vi "Close.vi"(8 "error in":errorcluster, 11 "lia host in":refnum<class "LIA Host Interface.lvclass">) -> (0 "error out":errorcluster, 3 "lia host out":refnum<class "LIA Host Interface.lvclass">)   [LabVIEW 2017, in "LIA Host Interface.lvclass"]
uses:
  LIA Host Interface.lvclass
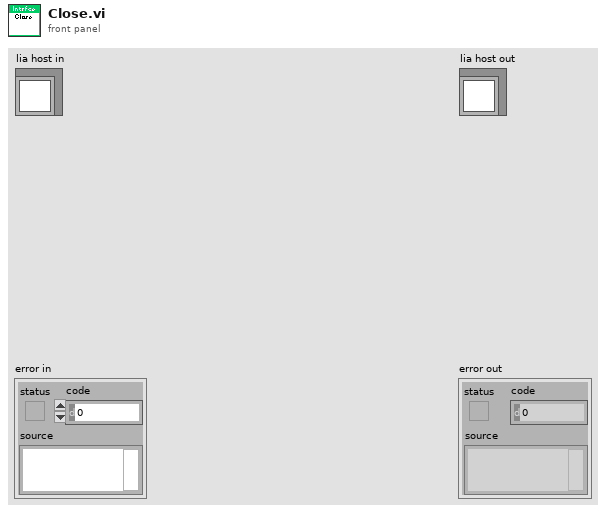
[diagram p1: front panel]
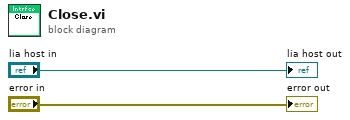
[diagram p0: block diagram]
diagram:
  "error out" <- "error in"
  "lia host out" <- "lia host in"
